vi "Periodic Tasks.vi"(8 "error in":errorcluster) -> ()   [LabVIEW 2013]
doc: "This VI runs in parallel to other tasks. It can contain as many user-defined periodic loops as you need. These can carry out PID or other sorts of timed response."
uses:
  <vilib>/Rock Robotics/SystemInterfaces/Utilities/FPGA_UtilitiesLED Source.ctl
  <vilib>/Rock Robotics/SystemInterfaces/Utilities/FPGA_UtilitiesLED State.ctl
  Robot Global Data.vi
panel:
  out "Distance":dbl
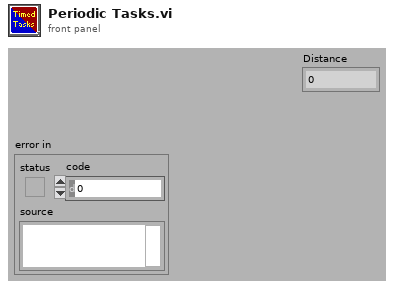
[diagram p1: front panel]
types:
  T1 = typedef "WPI_AnalogChannelDevRef.ctl" = cluster{"DevStatus":errorcluster, "Analog Module":T2, "Analog Channel":T3}
  T2 = typedef "FPGA_TypedefAnalogModule.ctl" = enum16{"Analog Module 1", "Analog Module 2"}
  T3 = typedef "FPGA_AIChannel.ctl" = enum8{"AI 1", "AI 2", "AI 3", "AI 4", "AI 5", "AI 6", "AI 7", "AI 8", "Invalid"}
  T4 = typedef "WPI_DigitalInputDevRef.ctl" = cluster{"DevStatus":errorcluster, "DIO Channel":T5, "Digital Module":T6}
  T5 = typedef "FPGA_DIOChannel.ctl" = enum8{"DIO 1", "DIO 2", "DIO 3", "DIO 4", "DIO 5", "DIO 6", "DIO 7", "DIO 8", "DIO 9", "DIO 10", "DIO 11", "DIO 12", "DIO 13", "DIO 14", "Invalid"}
  T6 = typedef "FPGA_TypedefDigitalModule.ctl" = enum16{"Digital Module 1", "Digital Module 2"}
  T7 = cluster{"Winch Desired Location":dbl, "Winch Desired Location 2":dbl, "Winch Desired Location 3":dbl}
  T8 = typedef "WPI_EncoderDevRef.ctl" = cluster{"DevStatus":errorcluster, "EncoderIndex":T9, "CounterIndex":T10, "DistancePerCount":dbl, "Decoding Type":T11}
  T9 = typedef "FPGA_EncoderIdx.ctl" = enum8{"Enc 0", "Enc 1", "Enc 2", "Enc 3", "Invalid"}
  T10 = typedef "FPGA_CounterCtrSystemIndex.ctl" = enum8{"Ctr 0", "Ctr 1", "Ctr 2", "Ctr 3", "Ctr 4", "Ctr 5", "Ctr 6", "Ctr 7", "Invalid"}
  T11 = typedef "WPI_EncoderType.ctl" = enum16{"1x", "2x", "4x"}
  T12 = typedef "FPGA_UtilitiesLED State.ctl" = enum16{"Off", "On", "Toggle"}
  T13 = typedef "FPGA_UtilitiesLED Source.ctl" = enum16{"User LED", "FPGA LED"}
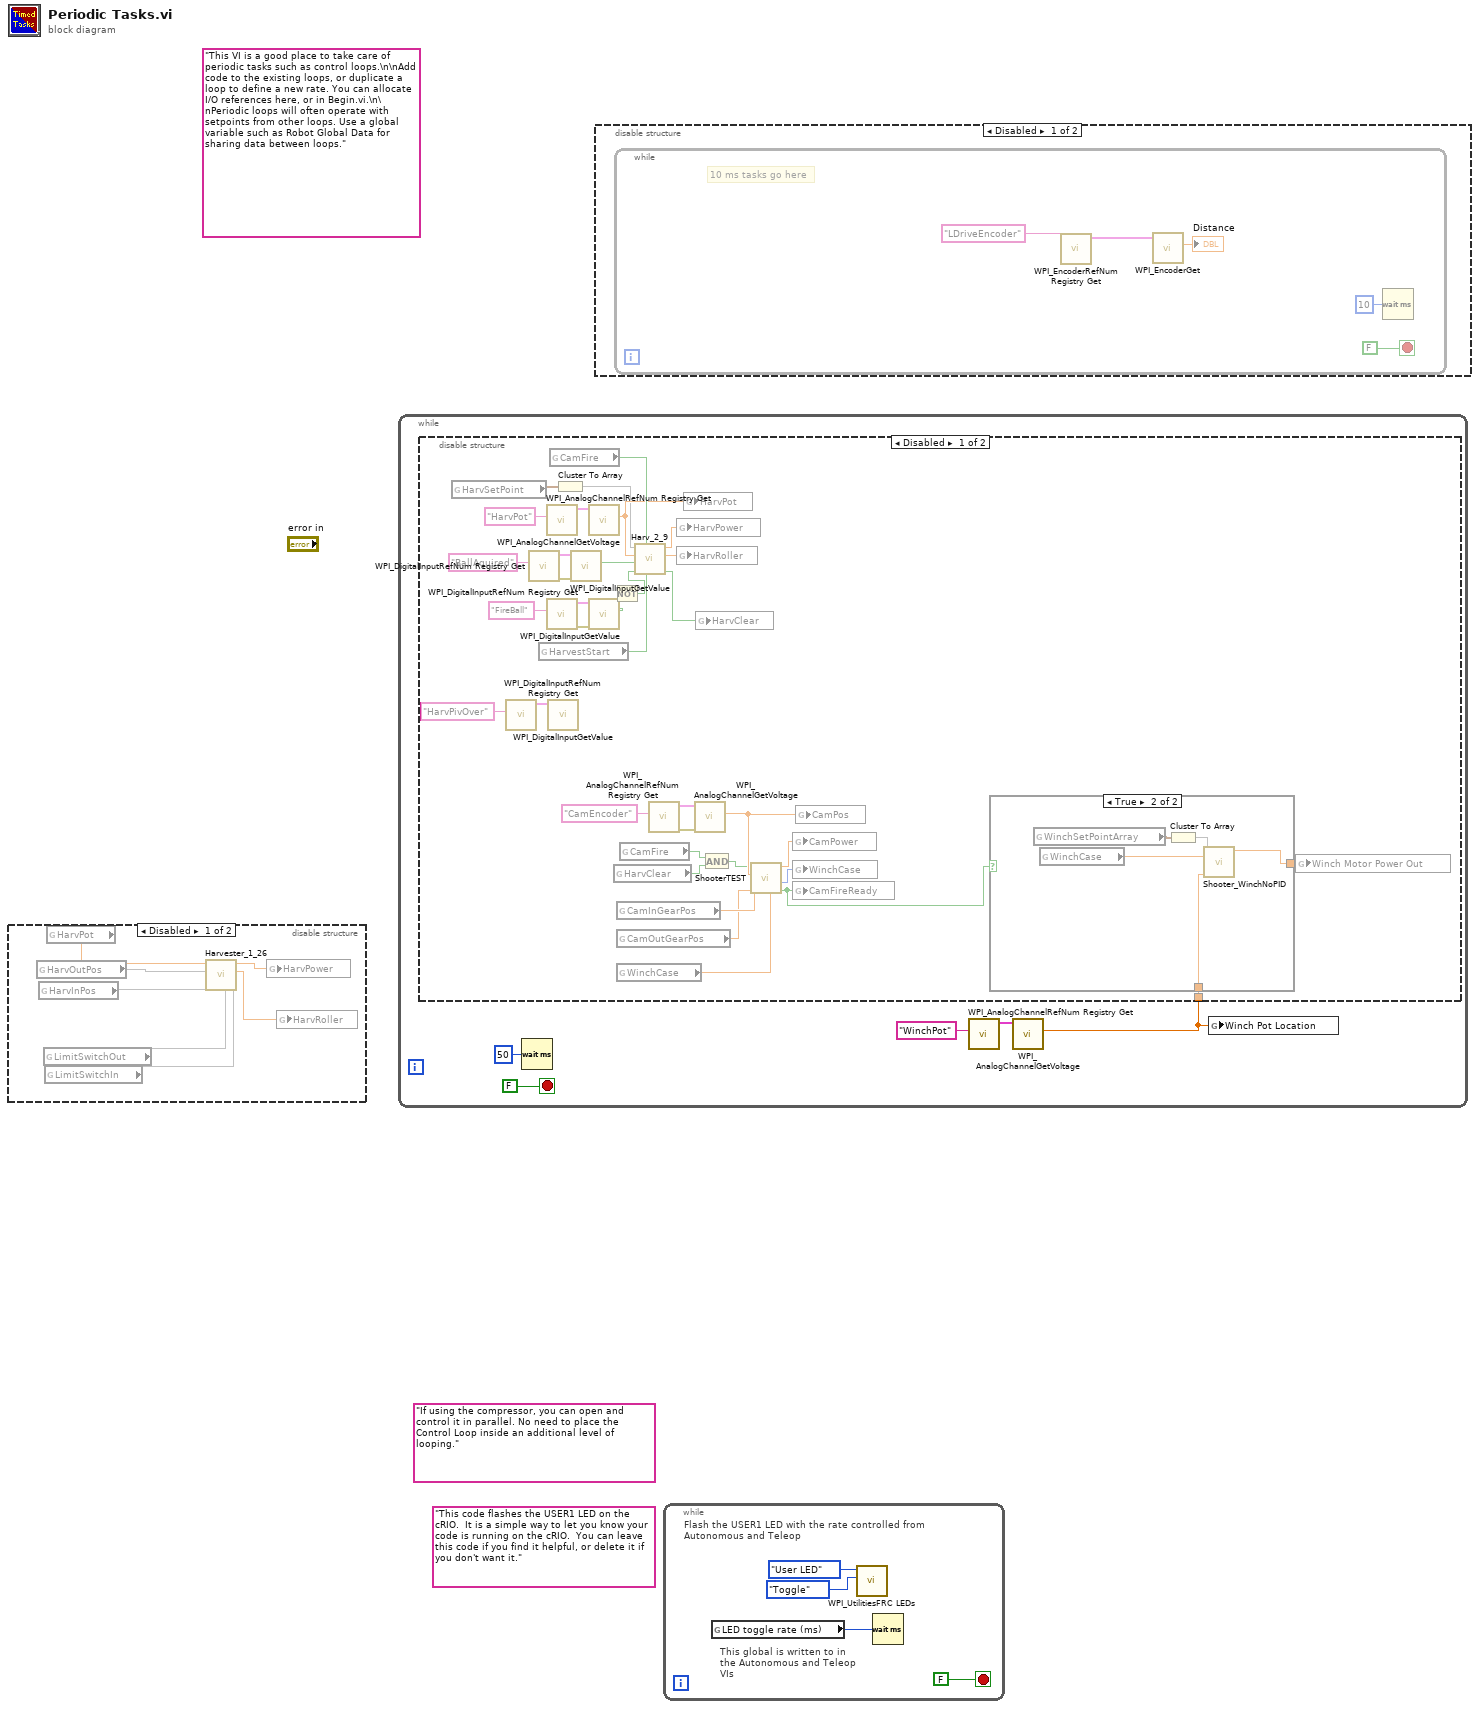
[diagram p0: block diagram]
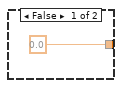
[diagram p4: hidden frame]
diagram:
  (unwired) "If using the compressor, you can open and control it in parallel. No need to place the Control Loop inside an additional level of looping."
  (unwired) "This code flashes the USER1 LED on the cRIO.  It is a simple way to let you know your code is running on the cRIO.  You can leave this code if you find it helpful, or delete it if you don't want it."
  (unwired) "This VI is a good place to take care of periodic tasks such as control loops.\n\nAdd code to the existing loops, or duplicate a loop to define a new rate. You can allocate I/O references here, or in Begin.vi.\n\nPeriodic loops will often operate with setpoints from other loops. Use a global variable such as Robot Global Data for sharing data between loops."
  n1 = disable-structure shown="Disabled" {
    frame Disabled {
      n2 = global read "Robot Global Data.vi" "HarvOutPos"() -> (w6)
      n3 = global read "Robot Global Data.vi" "HarvInPos"() -> (w5)
      n4 = global read "Robot Global Data.vi" "LimitSwitchOut"() -> (w4)
      n5 = global read "Robot Global Data.vi" "LimitSwitchIn"() -> (w3)
      n6 = global read "Robot Global Data.vi" "HarvPot"() -> (w7:dbl)
      n7 = call "Harvester_1_26.vi"("LimitSwitchIn"=w3, "LimitSwitchOut"=w4, "HarvInPos"=w5, "HarvOutPos"=w6, "HarvPot"=w7) -> ("HarvRoller"=w2:dbl, "HarvPower"=w1:dbl)  [unwired: 5 in]
      n8 = global write "Robot Global Data.vi" "HarvPower"(w1) -> ()
      n9 = global write "Robot Global Data.vi" "HarvRoller"(w2) -> ()
    }
    frame Enabled {
    }
  }
  n10 = while {
    stop <- FALSE stop-if-true
    n11 = Wait (ms)(milliseconds to wait=u32 50) -> ()  [unwired: 1 out]
    n12 = call <vilib>:"WPI_AnalogChannelRefNum Registry Get.vi"("refnum name"="WinchPot") -> ("AIDeviceRef"=w9:T1)  [unwired: 9 in, 1 out]
    n13 = call <vilib>:"WPI_AnalogChannelGetVoltage.vi"("AIDeviceRef"=w9) -> ("Voltage"=w8:dbl)  [unwired: 8 in, 2 out]
    n14 = disable-structure shown="Disabled" {
      disable-tunnel: w8 -> [w26 _]
      frame Disabled {
        n15 = global read "Robot Global Data.vi" "HarvSetPoint"() -> (w29:cluster{"Out":dbl, "In":dbl, "Clear":dbl})
        n16 = call <vilib>:"WPI_DigitalInputRefNum Registry Get.vi"("refnum name"="HarvPivOver") -> ("DigitalInputDevRef"=w31:T4)  [unwired: 9 in, 1 out]
        n17 = call <vilib>:"WPI_DigitalInputRefNum Registry Get.vi"("refnum name"="BallAquired") -> ("error out"=w48:errorcluster, "DigitalInputDevRef"=w47:T4)  [unwired: 9 in]
        n18 = global read "Robot Global Data.vi" "HarvestStart"() -> (w37:bool)
        n19 = call <vilib>:"WPI_AnalogChannelRefNum Registry Get.vi"("refnum name"="HarvPot") -> ("AIDeviceRef"=w43:T1)  [unwired: 9 in, 1 out]
        n20 = call <vilib>:"WPI_DigitalInputRefNum Registry Get.vi"("refnum name"="FireBall") -> ("error out"=w39:errorcluster, "DigitalInputDevRef"=w40:T4)  [unwired: 9 in]
        n21 = call <vilib>:"WPI_DigitalInputGetValue.vi"("DigitalInputDevRef"=w31) -> ()  [unwired: 8 in, 3 out]
        n22 = global read "Robot Global Data.vi" "CamFire"() -> (w38:bool)
        n23 = Cluster To Array(cluster=w29) -> (array=w28:dbl[])
        n24 = call <vilib>:"WPI_DigitalInputGetValue.vi"("error in (no error)"=w48, "DigitalInputDevRef"=w47) -> ("Value"=w33:bool)  [unwired: 7 in, 2 out]
        n25 = call <vilib>:"WPI_AnalogChannelGetVoltage.vi"("AIDeviceRef"=w43) -> ("Voltage"=w36:dbl)  [unwired: 8 in, 2 out]
        n26 = call <vilib>:"WPI_DigitalInputGetValue.vi"("error in (no error)"=w39, "DigitalInputDevRef"=w40) -> ("Value"=w35:bool)  [unwired: 7 in, 2 out]
        n27 = Not(x=w35) -> (.not. x?=w32:bool)
        n28 = global read "Robot Global Data.vi" "HarvClear"() -> (w17:bool)
        n29 = global read "Robot Global Data.vi" "CamInGearPos"() -> (w25:dbl)
        n30 = global read "Robot Global Data.vi" "CamOutGearPos"() -> (w24:dbl)
        n31 = global read "Robot Global Data.vi" "WinchCase"() -> (w18:dbl)
        n32 = global read "Robot Global Data.vi" "CamFire"() -> (w16:bool)
        n33 = call "Harv_2_9.vi"("Harvest"=w37, "Fire"=w38, "FireBallSen"=w32, "BallAcquired"=w33, "HarvPot"=w36, "HarvSetpoints"=w28) -> ("HarvCleared"=w34:bool, "HarvRoller"=w44:dbl, "HarvPower"=w45:dbl)  [unwired: 3 in]
        n34 = call <vilib>:"WPI_AnalogChannelRefNum Registry Get.vi"("refnum name"="CamEncoder") -> ("error out"=w22:errorcluster, "AIDeviceRef"=w21:T1)  [unwired: 9 in]
        n35 = global write "Robot Global Data.vi" "HarvPower"(w45) -> ()
        n36 = global write "Robot Global Data.vi" "HarvRoller"(w44) -> ()
        n37 = global write "Robot Global Data.vi" "HarvPot"(w36) -> ()
        n38 = call <vilib>:"WPI_AnalogChannelGetVoltage.vi"("error in (no error)"=w22, "AIDeviceRef"=w21) -> ("Voltage"=w20:dbl)  [unwired: 7 in, 2 out]
        n39 = global write "Robot Global Data.vi" "HarvClear"(w34) -> ()
        n40 = And(x=w16, y=w17) -> (x .and. y?=w15:bool)
        n41 = call "ShooterTEST.vi"("WinchCaseIn"=w18, "OutGearPos"=w24, "InGearPos"=w25, "Pot"=w20, "Fire"=w15) -> ("There?"=w13:bool, "WinchCase"=w19:i32, "Power"=w14:dbl)  [unwired: 4 in]
        n42 = global write "Robot Global Data.vi" "CamPower"(w14) -> ()
        n43 = global write "Robot Global Data.vi" "WinchCase"(w19) -> ()
        n44 = global write "Robot Global Data.vi" "CamFireReady"(w13) -> ()
        n45 = global write "Robot Global Data.vi" "CamPos"(w20) -> ()
        n46 = case shown="True" w13 {
          tunnel: [0.0 ("Winch Motor Power Out") w50] -> w27
          tunnel: w26 -> [_ w51]
          frame False {
          }
          frame True {
            n47 = global read "Robot Global Data.vi" "WinchSetPointArray"() -> (w53:T7)
            n48 = global read "Robot Global Data.vi" "WinchCase"() -> (w54:dbl)
            n49 = Cluster To Array(cluster=w53) -> (array=w52:dbl[])
            n50 = call "Shooter_WinchNoPID.vi"("Winch Pot Location"=w51, "selectedCase"=w54, "SetPointArray"=w52) -> ("Winch Motor Power Out"=w50:dbl)  [unwired: 8 in]
          }
        }
        n51 = global write "Robot Global Data.vi" "Winch Motor Power Out"(w27) -> ()
      }
      frame Enabled {
      }
    }
    n52 = global write "Robot Global Data.vi" "Winch Pot Location"(w8) -> ()
  }
  n53 = disable-structure shown="Disabled" {
    frame Disabled {
      n54 = while {
        stop <- FALSE stop-if-true
        # "10 ms tasks go here"
        n55 = call <vilib>:"WPI_EncoderRefNum Registry Get.vi"("refnum name"="LDriveEncoder") -> ("EncoderDevRef"=w55:T8)  [unwired: 9 in, 1 out]
        n56 = call <vilib>:"WPI_EncoderGet.vi"("EncoderDevRef"=w55) -> ("Distance"=→"Distance":dbl)  [unwired: 5 in, 5 out]
        n57 = Wait (ms)(milliseconds to wait=u32 10) -> ()  [unwired: 1 out]
      }
    }
    frame Enabled {
    }
  }
  n58 = while {
    stop <- FALSE stop-if-true
    # "This global is written to in the Autonomous and Teleop VIs"
    # "Flash the USER1 LED with the rate controlled from Autonomous and Teleop"
    n59 = global read "Robot Global Data.vi" "LED toggle rate (ms)"() -> (w60:u32)
    n60 = call <vilib>:"WPI_UtilitiesFRC LEDs.vi"("State"=FPGA_UtilitiesLED_State."Toggle", "LED Type"=FPGA_UtilitiesLED_Source."User LED") -> ()  [unwired: 1 in, 9 out]
    n61 = Wait (ms)(milliseconds to wait=w60) -> ()  [unwired: 1 out]
  }
